vi "Merge Sort 2D Coordinate Arrays.vi"(0 "2D Coordinate Array A":cluster{"x1":dbl, "x2":dbl}[](array[cluster]), 1 "Ignore Duplicates? (F)":bool, 3 "2D Coordinate Array B":cluster{"x1":dbl, "x2":dbl}[](array[cluster])) -> (6 "Sorted 2D Coordinate Array":cluster{"x1":dbl, "x2":dbl}[](array[cluster]))   [LabVIEW 2013]
panel:
  out "A Index":i32
  out "B Index":i32
  out "B Count":i32
  out "A Count":i32
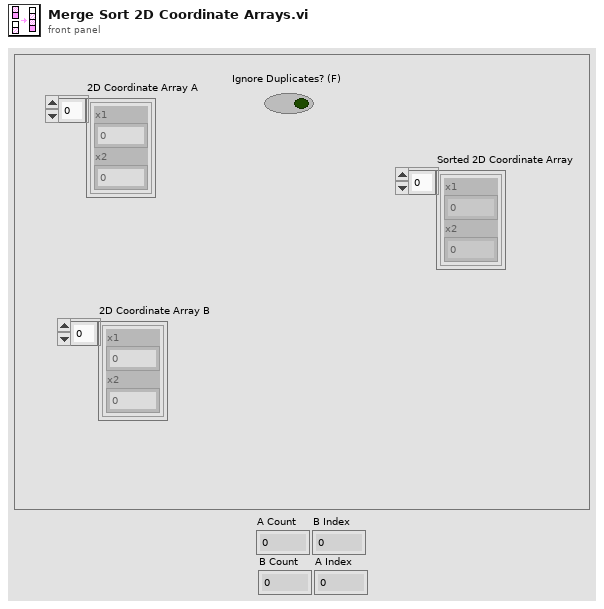
[diagram p1: front panel]
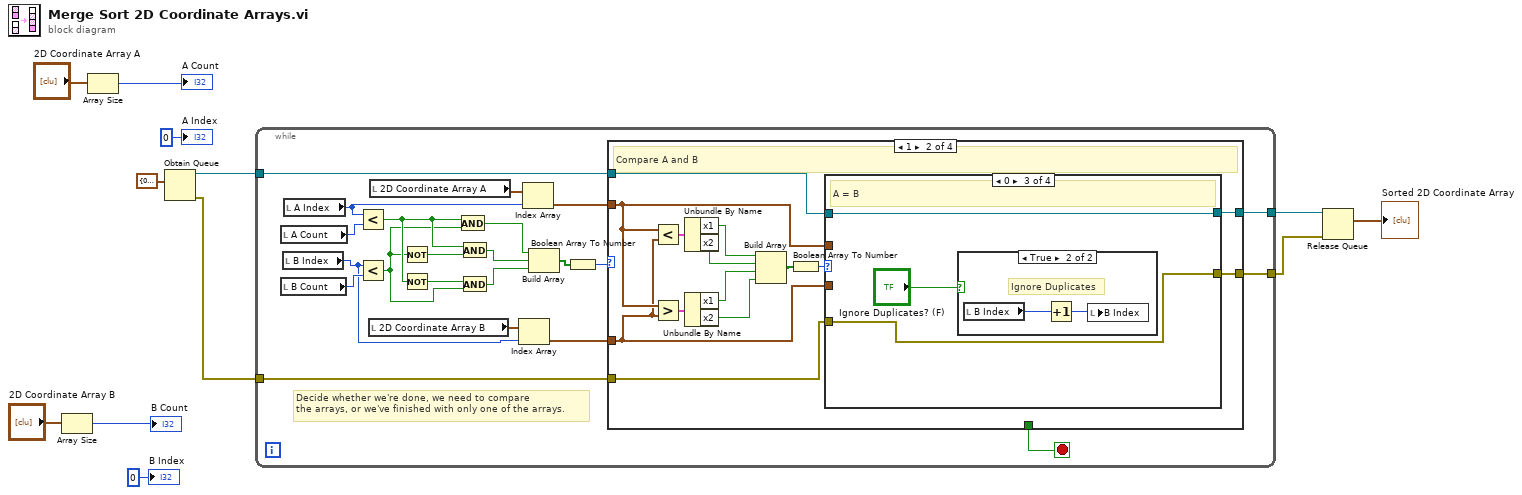
[diagram p0: block diagram]
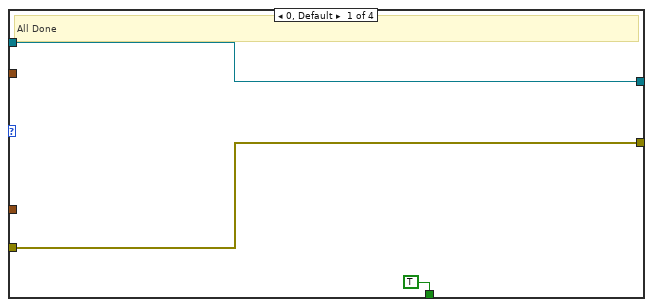
[diagram p2: hidden frame]
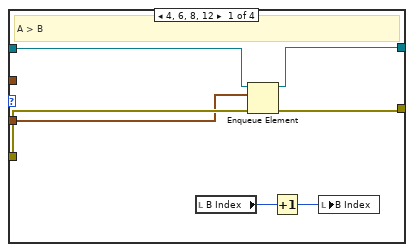
[diagram p3: hidden frame]
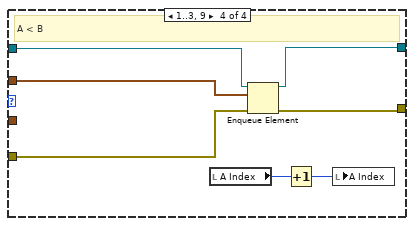
[diagram p6: hidden frame]
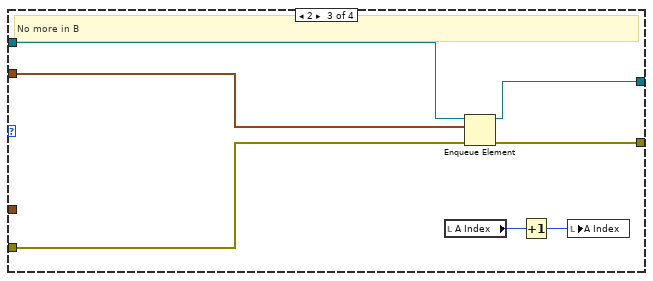
[diagram p7: hidden frame]
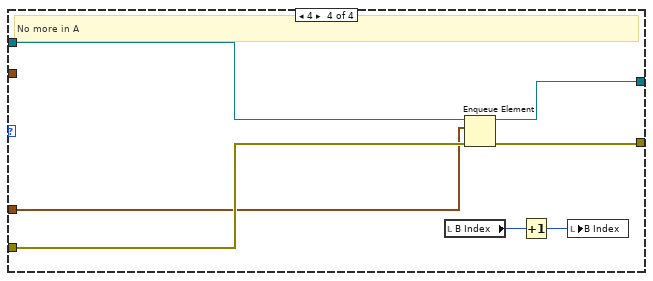
[diagram p8: hidden frame]
diagram:
  n1 = Array Size(array="2D Coordinate Array B") -> (size(s)=→"B Count":i32)
  n2 = Array Size(array="2D Coordinate Array A") -> (size(s)=→"A Count":i32)
  n3 = Obtain Queue(element data type=cluster{"x1":dbl, "x2":dbl} {"x1"=0.0, "x2"=0.0} ("2D Coordinate")) -> (queue out=w11:refnum<queue>, error out=w10:errorcluster)  [unwired: 4 in, 1 out]
  n4 = while {
    tunnel: w11 -> [w23]
    tunnel: [w22] -> w3
    tunnel: [w21] -> w12
    tunnel: w10 -> [w20]
    stop <- w13 stop-if-true
    # "Decide whether we're done, we need to compare\nthe arrays, or we've finished with only one of the arrays."
    n5 = local read "A Count"() -> (w34:i32)
    n6 = local read "B Count"() -> (w33:i32)
    n7 = local read "B Index"() -> (w16:i32)
    n8 = local read "A Index"() -> (w18:i32)
    n9 = Less?(x=w18, y=w34) -> (x < y?=w30:bool)
    n10 = Less?(x=w16, y=w33) -> (x < y?=w29:bool)
    n11 = local read "2D Coordinate Array B"() -> (w17:cluster{"x1":dbl, "x2":dbl}[])
    n12 = local read "2D Coordinate Array A"() -> (w19:cluster{"x1":dbl, "x2":dbl}[])
    n13 = Not(x=w29) -> (.not. x?=w27:bool)
    n14 = Not(x=w30) -> (.not. x?=w26:bool)
    n15 = And(x=w30, y=w29) -> (x .and. y?=w32:bool)
    n16 = And(x=w30, y=w27) -> (x .and. y?=w31:bool)
    n17 = And(x=w26, y=w29) -> (x .and. y?=w28:bool)
    n18 = Index Array(array=w17, index=w16) -> (element=w15:cluster{"x1":dbl, "x2":dbl})
    n19 = Index Array(array=w19, index=w18) -> (element=w14:cluster{"x1":dbl, "x2":dbl})
    n20 = Build Array(w32, w31, w28) -> (w25:bool[])
    n21 = Boolean Array To Number(Boolean array=w25) -> (number=w24:u32)
    n22 = case shown="1" w24 {
      tunnel: w23 -> [w37 w51 w79 w86]
      tunnel: w14 -> [_ w45 w77 _]
      tunnel: w15 -> [_ w44 _ w84]
      tunnel: w20 -> [w36 w46 w78 w85]
      tunnel: [w36 w50 w75 w82] -> w22
      tunnel: [w37 w49 w76 w83] -> w21
      tunnel: [TRUE _ _ _] -> w13
      frame 0, Default {
        # "All Done"
      }
      frame 1 {
        # "Compare A and B"
        n23 = Less?(x=w45, y=w44) -> (x < y?=w43:cluster{"x1":bool, "x2":bool})
        n24 = Greater?(x=w45, y=w44) -> (0:w42:cluster{"x1":bool, "x2":bool})
        n25 = Unbundle By Name(w43) -> ("x1"=w41:bool, "x2"=w40:bool)
        n26 = Unbundle By Name(w42) -> ("x1"=w39:bool, "x2"=w38:bool)
        n27 = Build Array(w41, w40, w39, w38) -> (w48:bool[])
        n28 = Boolean Array To Number(Boolean array=w48) -> (number=w47:u32)
        n29 = case shown="0" w47 {
          tunnel: w51 -> [w58 w60 w61 w72]
          tunnel: w45 -> [_ _ _ w71]
          tunnel: w44 -> [w52 _ _ _]
          tunnel: w46 -> [w57 w59 w62 w70]
          tunnel: [w55 w59 w62 w68] -> w50
          tunnel: [w56 w60 w61 w69] -> w49
          frame 4, 6, 8, 12 {
            # "A > B"
            n30 = local read "B Index"() -> (w53:i32)
            n31 = Enqueue Element(queue=w58, element=w52, error in (no error)=w57) -> (queue out=w56:refnum<queue>, error out=w55:errorcluster)  [unwired: 1 in, 1 out]
            n32 = Increment(x=w53) -> (x+1=w54:i32)
            n33 = local write "B Index"(w54) -> ()
          }
          frame Default {
            # "Shouldn't happen"
          }
          frame 0 {
            # "A = B"
            n34 = case shown="True" "Ignore Duplicates? (F)" {
              frame False {
              }
              frame True {
                # "Ignore Duplicates"
                n35 = local read "B Index"() -> (w65:i32)
                n36 = Increment(x=w65) -> (x+1=w64:i32)
                n37 = local write "B Index"(w64) -> ()
              }
            }
          }
          frame 1..3, 9 {
            # "A < B"
            n38 = local read "A Index"() -> (w66:i32)
            n39 = Enqueue Element(queue=w72, element=w71, error in (no error)=w70) -> (queue out=w69:refnum<queue>, error out=w68:errorcluster)  [unwired: 1 in, 1 out]
            n40 = Increment(x=w66) -> (x+1=w67:i32)
            n41 = local write "A Index"(w67) -> ()
          }
        }
      }
      frame 2 {
        # "No more in B"
        n42 = local read "A Index"() -> (w73:i32)
        n43 = Enqueue Element(queue=w79, element=w77, error in (no error)=w78) -> (queue out=w76:refnum<queue>, error out=w75:errorcluster)  [unwired: 1 in, 1 out]
        n44 = Increment(x=w73) -> (x+1=w74:i32)
        n45 = local write "A Index"(w74) -> ()
      }
      frame 4 {
        # "No more in A"
        n46 = local read "B Index"() -> (w80:i32)
        n47 = Enqueue Element(queue=w86, element=w84, error in (no error)=w85) -> (queue out=w83:refnum<queue>, error out=w82:errorcluster)  [unwired: 1 in, 1 out]
        n48 = Increment(x=w80) -> (x+1=w81:i32)
        n49 = local write "B Index"(w81) -> ()
      }
    }
  }
  n50 = Release Queue(queue=w12, error in (no error)=w3) -> (remaining elements=→"Sorted 2D Coordinate Array":cluster{"x1":dbl, "x2":dbl}[])  [unwired: 1 in, 2 out]
  "A Index" <- 0 ("A Index")
  "B Index" <- 0 ("B Index")
